vi "TEST_글로벌.vi"() -> ()   [LabVIEW 2020]
panel:
  out "불리언":bool
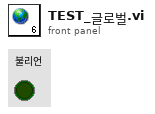
[diagram p1: front panel]
diagram:
